vi "Write Mux.vi"() -> ()   [LabVIEW 8.6]
uses:
  vi.lib/UeiDaq/UeiDaqConfigureTimingForSimpleIO.vi
  <libdir>/resource/objmgr/UeiDaq.rc
panel:
  in  "Break before make":bool
  out "ADC":dbl[](array[numeric])
  out "relayA":u32
  out "relayB":u32
  out "status":u32
  out "relayC":u32
  in  "Per channel Relay settings":cluster{"Channel":i32, "Relay":i32}[](array[cluster]) {"Relay" items=["All Off", "A", "B", "C"]}
  out "device name":string
  out "Number of channels":u32
  in  "Resource":string
  in  "stop":bool
  # "Mux Example"
  # "1/ Set the resource name -->"
  # "Device info"
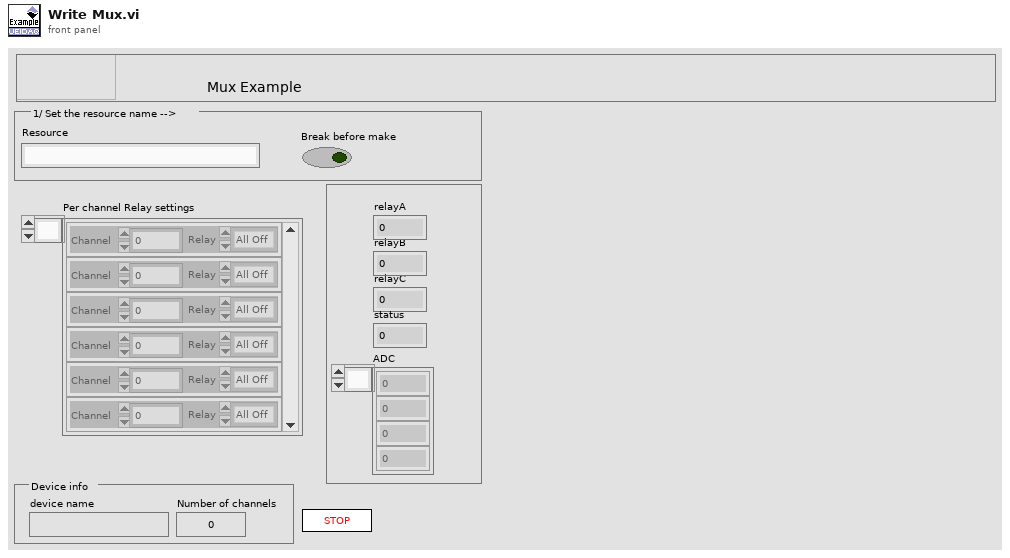
[diagram p1: front panel]
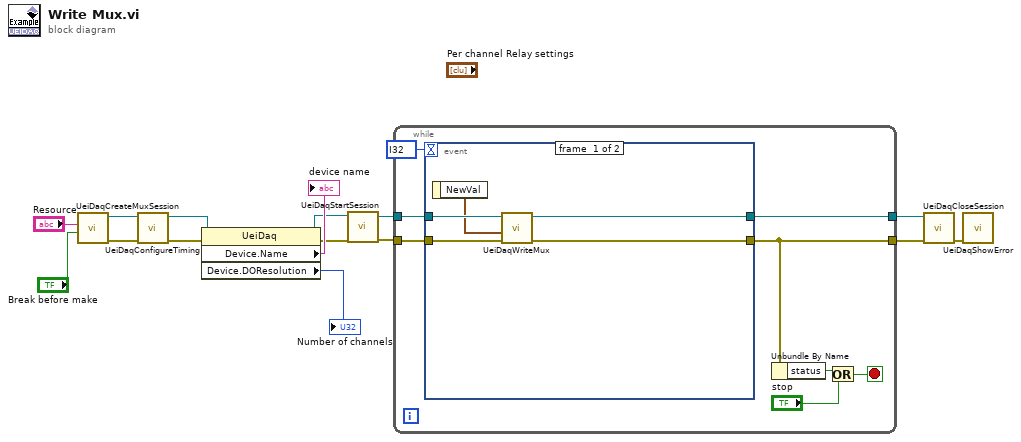
[diagram p0: block diagram]
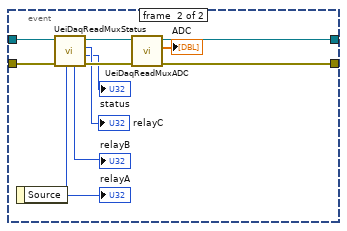
[diagram p2: hidden frame]
diagram:
  n1 = call "UeiDaqCreateMuxSession.vi"("Break before make"="Break before make", "Resource"="Resource") -> ("error out"=w13:errorcluster, "UeiDaq Refnum Out"=w14:refnum<k20>)  [unwired: 8 in]
  n2 = call-poly "UeiDaqConfigureTiming.vi"("error in (no error)"=w13, "UeiDaq Refnum In"=w14) -> ("error out"=w10:errorcluster, "UeiDaq Refnum Out"=w11:refnum<k20>)  [unwired: 1 in, 7 out]
  n3 = property class="UeiDaq"(reference=w11, error in=w10) -> (reference out=w1:refnum<k20>, error out=w2:errorcluster, "Device.Name"=→"device name":string, "Device.DOResolution"=→"Number of channels":u32)
  n4 = call <vilib>:"UeiDaqStartSession.vi"("error in (no error)"=w2, "UeiDaq Refnum In"=w1) -> ("error out"=w3:errorcluster, "UeiDaq Refnum Out"=w4:refnum<k20>)  [unwired: 8 in]
  n5 = while {
    tunnel: w4 -> [w19]
    tunnel: w3 -> [w20]
    tunnel: [w18] -> w9
    tunnel: [w17] -> w8
    stop <- w21 stop-if-true
    n6 = event shown="[1] Timeout" {
      selector: _ -> [_ _]
      dyn-events: _ -> [_ _]
      timeout: i32 ? -> [_ _]
      tunnel: w20 -> [w26 w38]
      tunnel: w19 -> [w28 w39]
      tunnel: [w25 w31] -> w18
      tunnel: [w24 w30] -> w17
      event #0 {
        n7 = event-data() -> ("NewVal"=w27:cluster{"Channel":i32, "Relay":i32}[])  [unwired: 1 in]
        n8 = call "UeiDaqWriteMux.vi"("error in (no error)"=w26, "Per channel relay configuration"=w27, "UeiDaq Refnum In"=w28) -> ("error out"=w25:errorcluster, "UeiDaq Refnum Out"=w24:refnum<k20>)  [unwired: 7 in]
      }
      event #1 {
        n9 = event-data() -> ()  [unwired: 1 in, 1 out]
        n10 = call "UeiDaqReadMuxStatus.vi"("error in (no error)"=w38, "UeiDaq Refnum In"=w39) -> ("error out"=w37:errorcluster, "status"=→"status":u32, "relayC"=→"relayC":u32, "UeiDaq Refnum Out"=w36:refnum<k20>, "relayB"=→"relayB":u32, "relayA"=→"relayA":u32)  [unwired: 4 in]
        n11 = call "UeiDaqReadMuxADC.vi"("UeiDaq Refnum In"=w36, "error in (no error)"=w37) -> ("UeiDaq Refnum Out"=w30:refnum<k20>, "ADC"=→"ADC":dbl[], "error out"=w31:errorcluster)  [unwired: 6 in]
      }
    }
    n12 = Unbundle By Name(w18) -> ("status"=w23:bool)
    n13 = Or(x=w23, y="stop") -> (x .or. y?=w21:bool)
  }
  n14 = call "UeiDaqCloseSession.vi"("error in (no error)"=w9, "UeiDaq Refnum In"=w8) -> ("error out"=w15:errorcluster)  [unwired: 1 in, 8 out]
  n15 = call "UeiDaqShowError.vi"("error in (no error)"=w15) -> ()  [unwired: 2 in, 9 out]
